vi "StringToI64[](cast).vi"(1 "String":string) -> (0 "I64[]":i64[](array[numeric]))   [LabVIEW 2012]
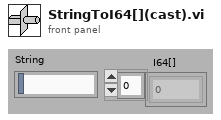
[diagram p1: front panel]
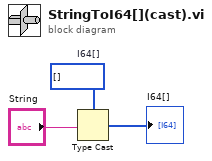
[diagram p0: block diagram]
diagram:
  w2 = i64[] []  # I64[]
  n1 = Type Cast(type=w2, x="String") -> (*(type *) &x=→"I64[]":i64[])
